vi "pruebaCONIMAQ.vi"() -> ()   [LabVIEW 2019]
uses:
  <vilib>/vision/Instrument.llb/QR Code Search Options.ctl
  <vilib>/vision/Instrument.llb/Demodulation Mode.ctl
  <vilib>/vision/Instrument.llb/Cell Sample Size.ctl
  <vilib>/vision/Instrument.llb/Cell Filter Mode.ctl
  <vilib>/vision/Instrument.llb/QR Code Description Options.ctl
  <vilib>/vision/Instrument.llb/Data Matrix Polarity.ctl
  <vilib>/vision/Instrument.llb/QR Code Model Type.ctl
  <vilib>/vision/NI_Vision_Development_Module.lvlib
panel:
  in  "DNVideoX":refnum<k7>(container)
  out "Datos_QR":string
  out "Error":errorcluster
  out "Imagen modificada":T1(plugin-control)
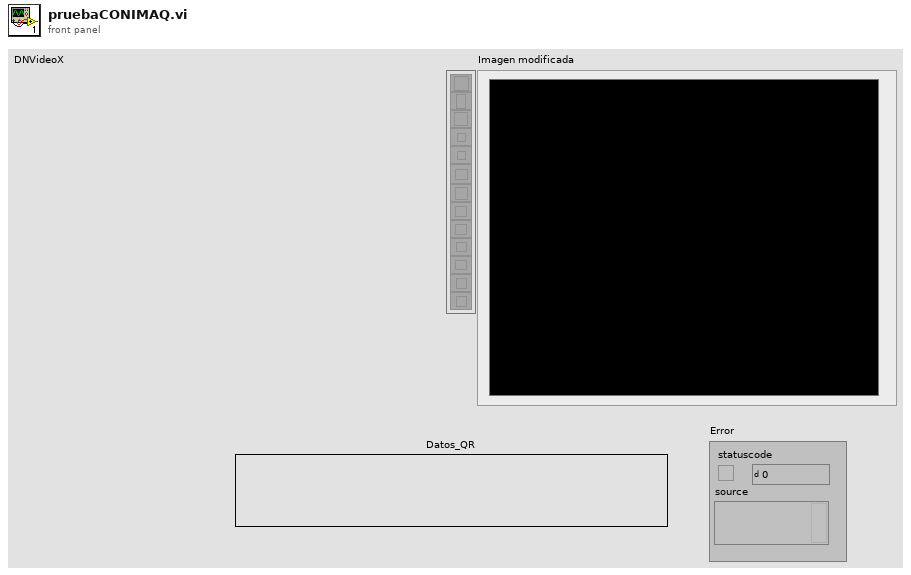
[diagram p1: front panel]
types:
  T1 = typedef "IMAQ Image.ctl" = refnum<image>
  T2 = typedef "QR Code Description Options.ctl" = cluster{"Matrix Size (cells)":i32, "Barcode Polarity":T3, "Mirror Mode":i32, "QR Model":T4}
  T3 = typedef "Data Matrix Polarity.ctl" = i32
  T4 = typedef "QR Code Model Type.ctl" = i32
  T5 = typedef "QR Code Search Options.ctl" = cluster{"Rotation Mode":enum32{"Unlimited", "0 Degrees", "90 Degrees", "180 Degrees", "270 Degrees"}, "Skip Location?":bool, "Edge Threshold":u32, "Demodulation Mode":T6, "Cell Sample Size":T7, "Cell Filter Mode":T8, "Skew Degrees Allowed":u32}
  T6 = typedef "Demodulation Mode.ctl" = i32
  T7 = typedef "Cell Sample Size.ctl" = i32
  T8 = typedef "Cell Filter Mode.ctl" = i32
  T9 = cluster{"Brightness":sgl, "Contrast":sgl, "Gamma":sgl}
  T10 = typedef "QR Code Report.ctl" = cluster{"Found?":bool, "Data":string, "Bounding Box":cluster{"x":sgl, "y":sgl}[], "Errors Corrected":u32, "Dimensions (Rows/Cols)":u32, "Version":u32, "QR Model":T4, "Stream Mode":T11, "Barcode Polarity":T3, "Mirrored?":bool, "Append Stream Position":u32, "Size of Append Stream":u32, "First EAN-128 ID":i32, "First Alternate Language ID":i32, "Append Stream ID":u32, "Minimum Edge Strength":u32, "Demodulation Mode":T6, "Cell Sample Size":T7, "Cell Filter Mode":T8}
  T11 = typedef "QR Code Stream Mode Type.ctl" = i32
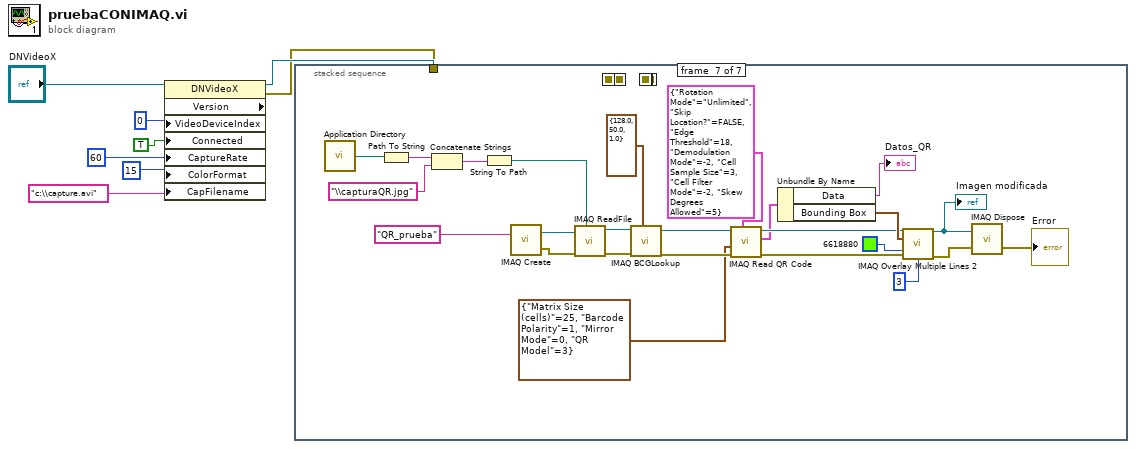
[diagram p0: block diagram]
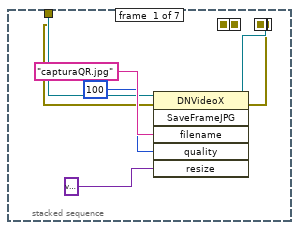
[diagram p2: hidden frame]
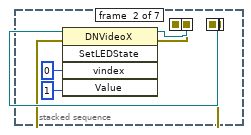
[diagram p3: hidden frame]
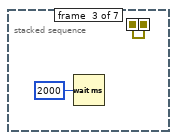
[diagram p4: hidden frame]
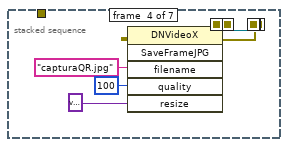
[diagram p5: hidden frame]
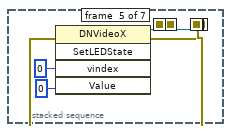
[diagram p6: hidden frame]
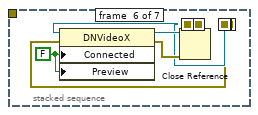
[diagram p7: hidden frame]
diagram:
  n1 = property class="DNVideoX" props=["Version", "VideoDeviceIndex", "Connected", "CaptureRate", "ColorFormat", "CapFilename"](reference="DNVideoX", "VideoDeviceIndex"=0, "Connected"=TRUE, "CaptureRate"=60 ("VideoDeviceIndex"), "ColorFormat"=15 ("VideoDeviceIndex"), "CapFilename"="c:\\capture.avi" ("default name")) -> (reference out=w3:refnum<k7>, error out=w2:errorcluster)  [unwired: 1 in, 1 out]
  n2 = stacked-sequence {
    seq-local: [w10 _ _ _ _ _ _] -> [_ w21 _ _ _ _ _]
    seq-local: [w9 _ _ _ _ _ _] -> [_ w20 _ _ _ _ _]
    seq-local: [_ w19 _ _ _ _ _] -> [_ _ w23 _ _ _ _]
    seq-local: [_ w18 _ _ _ _ _] -> [_ _ w22 _ _ _ _]
    seq-local: [_ _ w23 _ _ _ _] -> [_ _ _ w29 _ _ _]
    seq-local: [_ _ w22 _ _ _ _] -> [_ _ _ w25 _ _ _]
    seq-local: [_ _ _ w27 _ _ _] -> [_ _ _ _ w37 _ _]
    seq-local: [_ _ _ w26 _ _ _] -> [_ _ _ _ w36 _ _]
    seq-local: [_ _ _ _ w35 _ _] -> [_ _ _ _ _ w40 _]
    seq-local: [_ _ _ _ w34 _ _] -> [_ _ _ _ _ w39 _]
    tunnel: w3 -> [w12 _ _ _ _ _ _]
    tunnel: w2 -> [w11 _ _ _ _ _ _]
    frame #0 {
      n3 = invoke class="DNVideoX" method="SaveFrameJPG"(reference=w12, error in=w11, "filename"="capturaQR.jpg", "quality"=100, "resize"=variant) -> (reference out=w10:refnum<k7>, error out=w9:errorcluster)  [unwired: 1 in, 4 out]
    }
    frame #1 {
      n4 = invoke class="DNVideoX" method="SetLEDState"(reference=w21, error in=w20, "vindex"=0, "Value"=1) -> (reference out=w19:refnum<k7>, error out=w18:errorcluster)  [unwired: 1 in, 3 out]
    }
    frame #2 {
      n5 = Wait (ms)(milliseconds to wait=u32 2000) -> ()  [unwired: 1 out]
    }
    frame #3 {
      n6 = invoke class="DNVideoX" method="SaveFrameJPG"(reference=w29, error in=w25, "filename"="capturaQR.jpg", "quality"=100, "resize"=variant) -> (reference out=w27:refnum<k7>, error out=w26:errorcluster)  [unwired: 1 in, 4 out]
    }
    frame #4 {
      n7 = invoke class="DNVideoX" method="SetLEDState"(reference=w37, error in=w36, "vindex"=0, "Value"=0) -> (reference out=w35:refnum<k7>, error out=w34:errorcluster)  [unwired: 1 in, 3 out]
    }
    frame #5 {
      w38 = FALSE ("Connected")
      n8 = property class="DNVideoX"(reference=w40, error in=w39, "Connected"=w38, "Preview"=w38) -> (reference out=w41:refnum<k7>, error out=w42:errorcluster)
      n9 = Close Reference(reference=w41, error in (no error)=w42) -> ()  [unwired: 1 out]
    }
    frame #6 {
      n10 = call <vilib>:"Application Directory.vi"() -> ("Application Directory"=w48:path)
      n11 = Path To String(path=w48) -> (string=w51:string)
      n12 = Concatenate Strings(w51, "\\capturaQR.jpg" ("Image Name")) -> (w49:string)
      n13 = String To Path(string=w49) -> (path=w46:path)
      n14 = call "IMAQ Create"("Image Name"="QR_prueba") -> ("New Image"=w43:T1, "error out"=w44:errorcluster)  [unwired: 4 in]
      n15 = call "IMAQ ReadFile"("File Path"=w46, "error in (no error)"=w44, "Image"=w43) -> ("error out"=w65:errorcluster, "Image Out"=w53:T1)  [unwired: 4 in, 3 out]
      n16 = call "IMAQ BCGLookup"("Image Src"=w53, "BCG Values"=T9 {"Brightness"=128.0, "Contrast"=50.0, "Gamma"=1.0}, "error in (no error)"=w65) -> ("Image Dst Out"=w66:T1, "error out"=w67:errorcluster)  [unwired: 4 in]
      n17 = call "IMAQ Read QR Code"("QR Search Options"=T5 {"Rotation Mode"=enum."Unlimited", "Skip Location?"=FALSE, "Edge Threshold"=18, "Demodulation Mode"=-2, "Cell Sample Size"=3, "Cell Filter Mode"=-2, "Skew Degrees Allowed"=5}, "error in (no error)"=w67, "QR Description Options"=T2 {"Matrix Size (cells)"=25, "Barcode Polarity"=1, "Mirror Mode"=0, "QR Model"=3}, "Image"=w66) -> ("error out"=w63:errorcluster, "QR Code Report"=w58:T10, "Image (duplicate)"=w61:T1)  [unwired: 4 in, 1 out]
      n18 = Unbundle By Name(w58) -> ("Data"=→"Datos_QR":string, "Bounding Box"=w64:cluster{"x":sgl, "y":sgl}[])
      n19 = call "IMAQ Overlay Multiple Lines 2"("Image"=w61, "Line End Points"=w64, "Color"=u32 6618880, "error in (no error)"=w63, "Width"=u32 3) -> ("Image Out"=w52:T1, "error out"=w62:errorcluster)  [unwired: 9 in]
      "Imagen modificada" <- w52
      n20 = call "IMAQ Dispose"("Image"=w52, "error in (no error)"=w62) -> ("error out"=→"Error":errorcluster)  [unwired: 4 in]
    }
  }
